vi "Save VI State.vi"(8 "error in (no error)":errorcluster, 10 "state file path (<application path>\\<vi name>.state)":path, 11 "vi reference (caller VI)":refnum<vi>) -> (0 "error out":errorcluster)   [LabVIEW 2015, in "PL Utility.lvlib"]
doc: "Saves control and indicator values to binary file specified by <b>state file path</b> for the VI specified by <b>vi reference</b>."
uses:
  PL Utility.lvlib
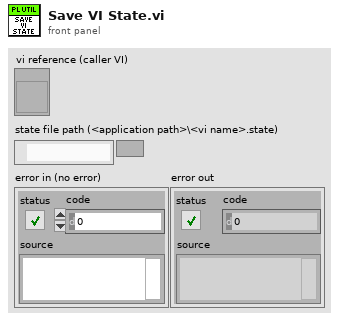
[diagram p1: front panel]
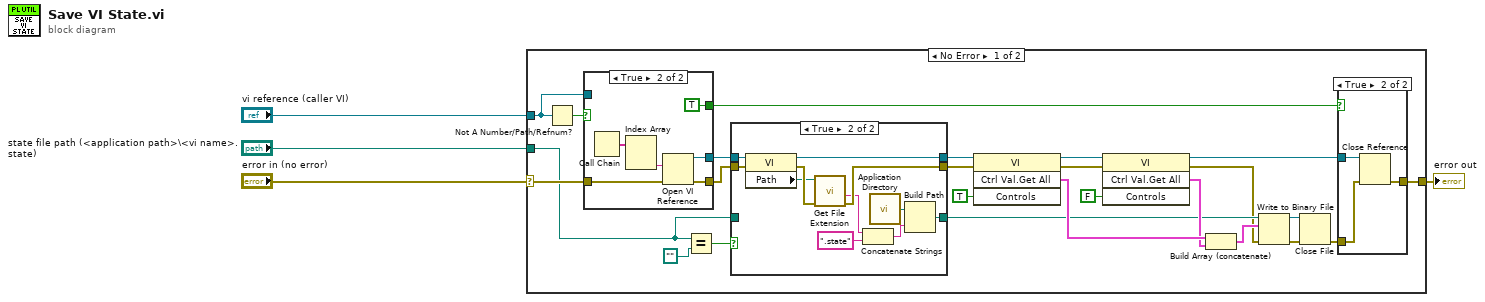
[diagram p0: block diagram]
diagram:
  n1 = case shown="No Error" "error in (no error)" {
    selector: "error in (no error)" -> [w27 w56]
    tunnel: [w13 w56] -> w3
    tunnel: "state file path (<application path>\\<vi name>.state)" -> [w22 _]
    tunnel: "vi reference (caller VI)" -> [w28 _]
    frame No Error {
      n2 = Not A Number/Path/Refnum?(number/path/refnum=w28) -> (NaN/Path/Refnum?=w29:bool)
      n3 = case shown="True" w29 {
        tunnel: w28 -> [w49 _]
        tunnel: [w49 w53] -> w26
        tunnel: w27 -> [w48 w52]
        tunnel: [w48 w51] -> w25
        tunnel: [_ TRUE] -> w14
        frame False {
        }
        frame True {
          n4 = Call Chain() -> (call chain=w55:string[])
          n5 = Index Array(array=w55) -> (element #2=w54:string)  [unwired: 2 in, 1 out]
          n6 = Open VI Reference(vi path=w54, error in (no error)=w52) -> (vi reference=w53:refnum<vi>, error out=w51:errorcluster)  [unwired: 4 in]
        }
      }
      n7 = Equal?(x=w22, y=path "") -> (x = y?=w23:bool)
      n8 = case shown="True" w23 {
        tunnel: w26 -> [w35 w47]
        tunnel: w25 -> [w34 w46]
        tunnel: w22 -> [w36 _]
        tunnel: [w36 w43] -> w9
        tunnel: [w35 w45] -> w19
        tunnel: [w34 w40] -> w10
        frame False {
        }
        frame True {
          n9 = property class="VI"(reference=w47, error in=w46) -> (reference out=w45:refnum<vi>, error out=w42:errorcluster, "Path"=w41:path)
          n10 = call <vilib>:"Get File Extension.vi"("error in (no error)"=w42, "file"=w41) -> ("error out"=w40:errorcluster, "filename without extension"=w38:string)  [unwired: 5 in, 3 out]
          n11 = Concatenate Strings(w38, ".state" ("string")) -> (w39:string)
          n12 = call <vilib>:"Application Directory.vi"() -> ("Application Directory"=w44:path)
          n13 = Build Path(base path=w44, name or relative path=w39) -> (appended path=w43:path)
        }
      }
      n14 = invoke class="VI" method="Ctrl Val.Get All"(reference=w19, error in=w10, "Controls"=TRUE) -> (reference out=w17:refnum<vi>, error out=w20:errorcluster, "Get All Control Values Variant"=w16:cluster{"Name":string, "Variant Data":variant}[])  [unwired: 1 in, 1 out]
      n15 = invoke class="VI" method="Ctrl Val.Get All"(reference=w17, error in=w20, "Controls"=FALSE) -> (reference out=w12:refnum<vi>, error out=w8:errorcluster, "Get All Control Values Variant"=w15:cluster{"Name":string, "Variant Data":variant}[])  [unwired: 1 in, 1 out]
      n16 = Build Array (concatenate)(w16, w15) -> (w11:cluster{"Name":string, "Variant Data":variant}[])
      n17 = Write to Binary File(file (use dialog)=w9, data=w11, error in=w8) -> (refnum out=w7:refnum<file>, error out=w6:errorcluster)  [unwired: 3 in, 1 out]
      n18 = Close File(refnum=w7, error in=w6) -> (error out=w5:errorcluster)  [unwired: 1 out]
      n19 = case shown="True" w14 {
        tunnel: w5 -> [w30 w31]
        tunnel: [w30 w32] -> w13
        tunnel: w12 -> [_ w33]
        frame False {
        }
        frame True {
          n20 = Close Reference(reference=w33, error in (no error)=w31) -> (error out=w32:errorcluster)
        }
      }
    }
    frame Error {
    }
  }
  "error out" <- w3
